vi "DisplayFilesToMerge.vi"(4 "Error In":errorcluster, 7 "MergeFileConfigIN":T1) -> (0 "Error Out":errorcluster, 1 "QualisysWaveform":waveform(dbl)[](graph), 2 "HBMWaveForms":waveform(dbl)[](graph), 3 "PCIWaveform":waveform(dbl)[](graph))   [LabVIEW 2017]
uses:
  DefDeType/MergeFileConfig.ctl
  DefDeType/WhichPath.ctl
panel:
  out "size(s)":i32
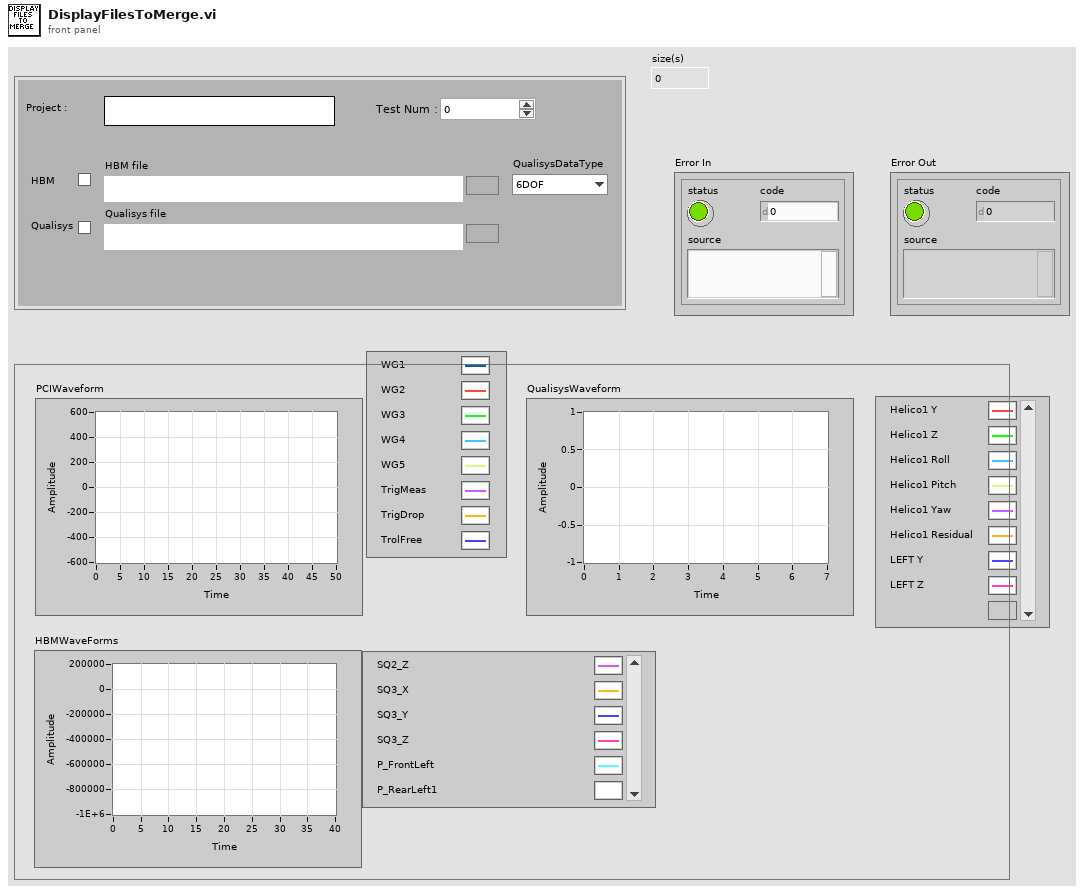
[diagram p1: front panel]
types:
  T1 = typedef "MergeFileConfig.ctl" = cluster{"Test Num : ":u32, "Project :":string, "Qualisys file":path, "HBM file":path, "QualisysDataType":enum16{"6DOF", "3DTracking", "6DOF + 3D"}, "Qualisys":bool, "HBM":bool}
  T2 = typedef "WhichPath.ctl" = enum16{"DossierProjet", "Config", "Meas", "MeasPCI", "MeasCRIO1", "MeasCRIO2", "MeasQualisys", "MeasHBM", "MeasTDMS", "Fig", "Res"}
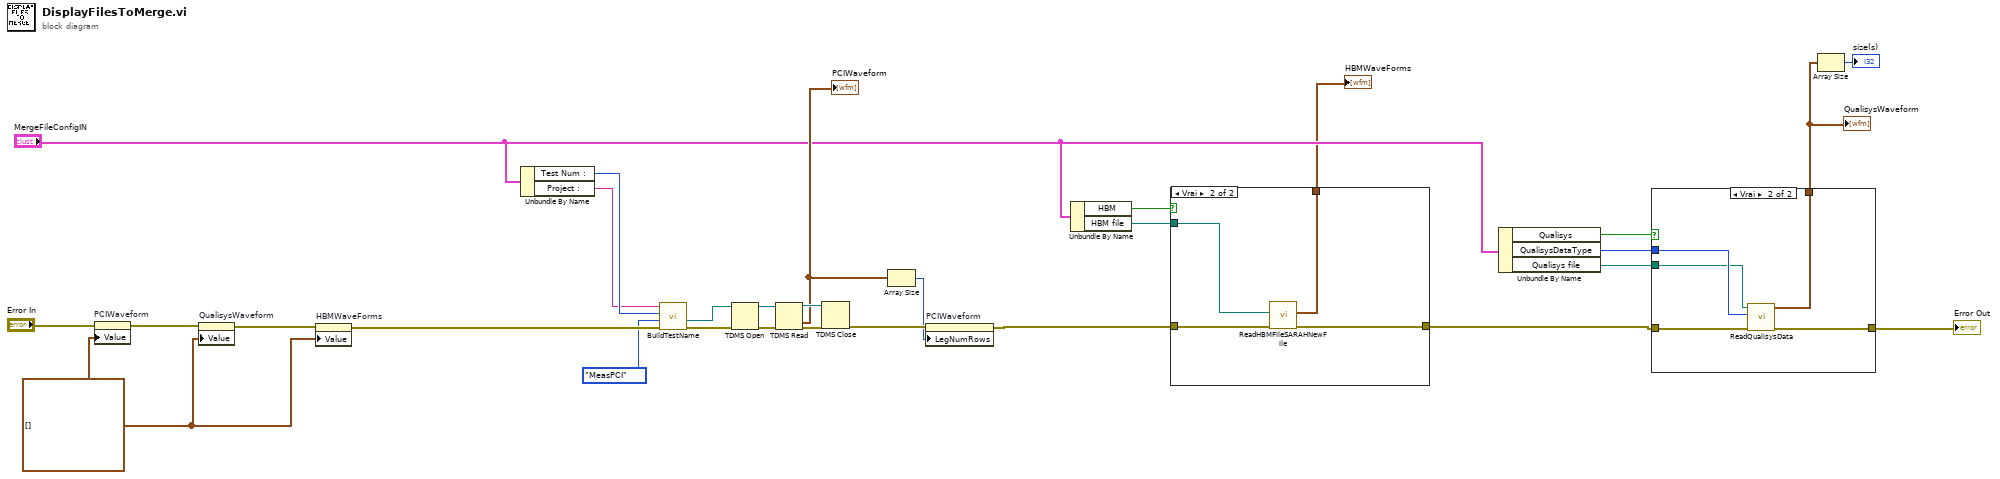
[diagram p0: block diagram]
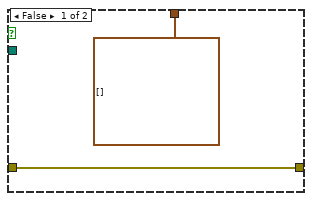
[diagram p2: hidden frame]
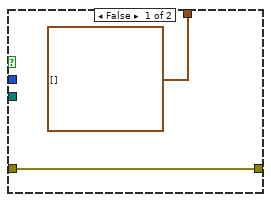
[diagram p3: hidden frame]
diagram:
  w26 = waveform(dbl)[] [] ("QualisysWaveforms")
  n1 = property on="PCIWaveform" class="GraphWF (strict)"(error in="Error In", "Value"=w26) -> (error out=w28:errorcluster)  [unwired: 1 in, 1 out]
  n2 = property on="QualisysWaveform" class="GraphWF (strict)"(error in=w28, "Value"=w26) -> (error out=w27:errorcluster)  [unwired: 1 in, 1 out]
  n3 = property on="HBMWaveForms" class="GraphWF (strict)"(error in=w27, "Value"=w26) -> (error out=w2:errorcluster)  [unwired: 1 in, 1 out]
  n4 = Unbundle By Name("MergeFileConfigIN") -> ("Test Num :"=w23:u32, "Project :"=w15:string)
  n5 = call "BuildTestName.vi"("entrée d'erreur"=w2, "WhichPath?"=WhichPath."MeasPCI", "NextTestNum"=w23, "NomProjet"=w15) -> ("sortie d'erreur"=w25:errorcluster, "cheminProchainFichier"=w24:path)  [unwired: 1 in, 2 out]
  n6 = TDMS Open(8:w25, 11:w24) -> (0:w21:errorcluster, 3:w22:refnum<k34>)  [unwired: 5 in]
  n7 = TDMS Read(0:w22, 11:w21) -> (4:w20:refnum<k34>, 10:w13:waveform(dbl)[], 15:w19:errorcluster)  [unwired: 6 in, 3 out]
  "PCIWaveform" <- w13
  n8 = TDMS Close(8:w19, 11:w20) -> (0:w14:errorcluster)  [unwired: 1 out]
  n9 = Array Size(array=w13) -> (size(s)=w12:i32)
  n10 = property on="PCIWaveform" class="GraphWF (strict)"(error in=w14, "LegNumRows"=w12) -> (error out=w8:errorcluster)  [unwired: 1 in, 1 out]
  n11 = Unbundle By Name("MergeFileConfigIN") -> ("HBM"=w6:bool, "HBM file"=w5:path)
  n12 = case shown="Vrai" w6 {
    tunnel: w8 -> [w31 w35]
    tunnel: [w31 w34] -> w7
    tunnel: w5 -> [_ w33]
    tunnel: [waveform(dbl)[] [] ("data") w32] -> w3
    frame False {
    }
    frame True {
      n13 = call "ReadHBMFileSARAHNewFile.vi"("error in (no error)"=w35, "file path"=w33) -> ("error out"=w34:errorcluster, "HBMWaveformsOut"=w32:waveform(dbl)[])  [unwired: 4 in]
    }
  }
  "HBMWaveForms" <- w3
  n14 = Unbundle By Name("MergeFileConfigIN") -> ("Qualisys"=w16:bool, "QualisysDataType"=w17:enum16{"6DOF", "3DTracking", "6DOF + 3D"}, "Qualisys file"=w18:path)
  n15 = case shown="Vrai" w16 {
    tunnel: [w37 w42] -> w4
    tunnel: w7 -> [w37 w38]
    tunnel: w17 -> [_ w41]
    tunnel: [waveform(dbl)[] [] ("QualisysWaveforms") w40] -> w11
    tunnel: w18 -> [_ w39]
    frame False {
    }
    frame True {
      n16 = call "ReadQualisysData.vi"("sortie d'erreur"=w38, "QualisysDataType"=w41, "QualisysFile"=w39) -> ("error out"=w42:errorcluster, "Waveform Graph"=w40:waveform(dbl)[])  [unwired: 3 in]
    }
  }
  "QualisysWaveform" <- w11
  "Error Out" <- w4
  n17 = Array Size(array=w11) -> (size(s)=→"size(s)":i32)
